vi "Set or Clear LVClass Default Menu.vi"(8 "error in (no error)":errorcluster, 10 "Name of .mnu file to set as Default Menu -- empty string to delete existing":string, 11 "LV Class in":refnum<vi>) -> (0 "error out":errorcluster, 3 "LV Class out":refnum<vi>)   [LabVIEW 2020]
doc: "This VI tags a LabVIEW class as having or not having (if you pass the empty string) a default palette menu. The default menu is the one that appears when you right click on a wire or terminal of that class type."
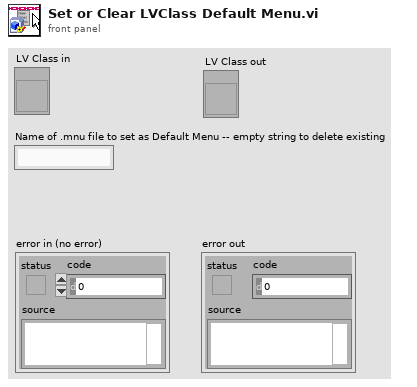
[diagram p1: front panel]
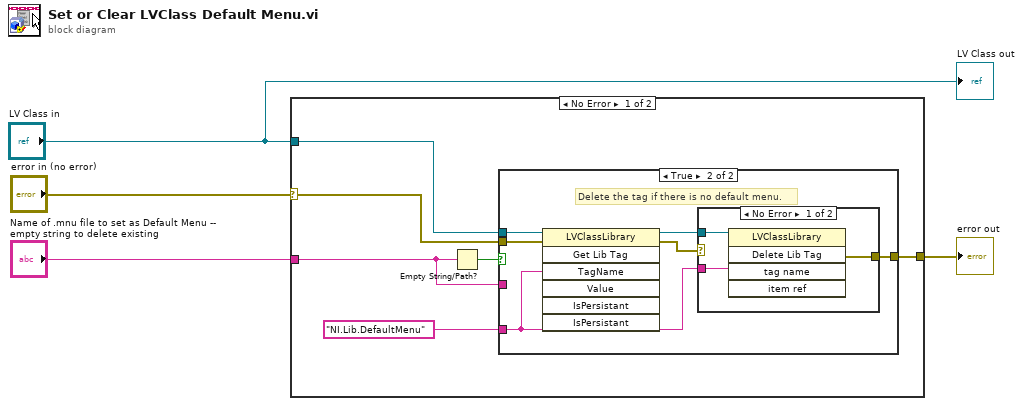
[diagram p0: block diagram]
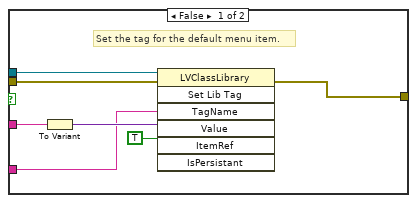
[diagram p2: hidden frame]
diagram:
  n1 = case shown="No Error" "error in (no error)" {
    selector: "error in (no error)" -> [w5 w27]
    tunnel: [w10 w27] -> w4
    tunnel: "Name of .mnu file to set as Default Menu -- empty string to delete existing" -> [w9 _]
    tunnel: "LV Class in" -> [w6 _]
    frame No Error {
      n2 = Empty String/Path?(string/path=w9) -> (empty?=w7:bool)
      n3 = case shown="True" w7 {
        tunnel: w5 -> [w15 w21]
        tunnel: w6 -> [w14 w22]
        tunnel: [w13 w23] -> w10
        tunnel: w9 -> [w12 _]
        tunnel: "NI.Lib.DefaultMenu" -> [w11 w18]
        frame False {
          # "Set the tag for the default menu item."
          n4 = To Variant(anything=w12) -> (Variant=w17:variant)
          n5 = invoke class="LVClassLibrary" method="Set Lib Tag"(reference=w14, error in=w15, "TagName"=w11, "Value"=w17, "ItemRef"=TRUE) -> (error out=w13:errorcluster)  [unwired: 2 in, 6 out]
        }
        frame True {
          # "Delete the tag if there is no default menu."
          n6 = invoke class="LVClassLibrary" method="Get Lib Tag"(reference=w22, error in=w21, "TagName"=w18) -> (reference out=w20:refnum<vi>, error out=w19:errorcluster)  [unwired: 4 in, 5 out]
          n7 = case shown="No Error" w19 {
            tunnel: [w26 _] -> w23
            tunnel: w20 -> [w25 _]
            tunnel: w18 -> [w24 _]
            frame No Error {
              n8 = invoke class="LVClassLibrary" method="Delete Lib Tag"(reference=w25, "tag name"=w24) -> (error out=w26:errorcluster)  [unwired: 3 in, 4 out]
            }
            frame Error {
              # "Do not propagate this\nerror. An error is thrown\nif the tag is missing."
            }
          }
        }
      }
    }
    frame Error {
    }
  }
  "error out" <- w4
  "LV Class out" <- "LV Class in"
